vi "UpdateRequestAlarm.vi"(8 "error in":errorcluster, 9 "Alarm":bool, 10 "RequestID":string) -> (0 "error out":errorcluster)   [LabVIEW 2015, in "DatabaseApi.lvlib"]
uses:
  DatabaseApi.lvlib
  TypeDef/Request/RequestsTableColumnNamesRing.ctl
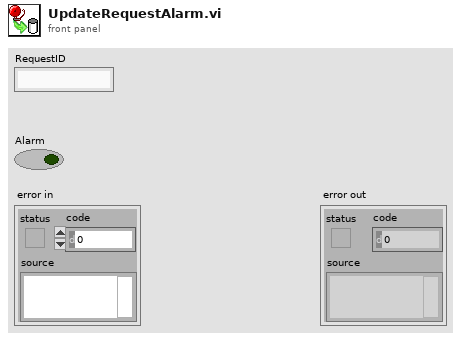
[diagram p1: front panel]
types:
  T1 = typedef "DatabaseApi.lvlib/RequestsTableColumnNamesRing.ctl" = enum16{"RequestID", "PersonnelType", "StartTime", "StartName", "AckTime", "AckName", "FulfilledTime", "FulfilledName", "Description", "Room Number", "Request Type", "Alarm"}
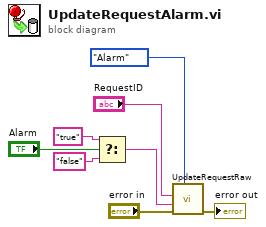
[diagram p0: block diagram]
diagram:
  n1 = Select(t="true", s="Alarm", f="false") -> (s? t:f=w1:string)
  n2 = call "UpdateRequestRaw.vi"("Data to update"=RequestsTableColumnNamesRing."Alarm", "error in"="error in", "data"=w1, "RequestID"="RequestID") -> ("error out"=→"error out":errorcluster)  [unwired: 7 in]
